vi "state name updater.vi"(1 "State Names":string[](array[string]), 2 "State Settings in":T1[][](array[typedef]) {"valve cycle time" min=0.2 step=0.1 format="%.2f"; "flow division"."5" min=0.0 max=1.0 step=0.01 format="%.3f"; "flow division"."4" min=0.0 max=1.0 step=0.01 format="%.3f"; "flow division"."3" min=0.0 max=1.0 step=0.01 format="%.3f"; "flow division"."2" min=0.0 max=1.0 step=0.01 format="%.3f"; "flow division"."1" min=0.0 max=1.0 step=0.01 format="%.3f"; "flow rate" format="%.3f"}) -> (0 "State Settings out":T1[][](array[typedef]) {"valve cycle time" min=0.2 step=0.1 format="%.2f"; "flow division"."5" min=0.0 max=1.0 step=0.01 format="%.3f"; "flow division"."4" min=0.0 max=1.0 step=0.01 format="%.3f"; "flow division"."3" min=0.0 max=1.0 step=0.01 format="%.3f"; "flow division"."2" min=0.0 max=1.0 step=0.01 format="%.3f"; "flow division"."1" min=0.0 max=1.0 step=0.01 format="%.3f"; "flow rate" format="%.3f"})   [LabVIEW 2012]
uses:
  State Setting.ctl
  Stamp/Switch settings vertical.ctl
  flow fraction.ctl
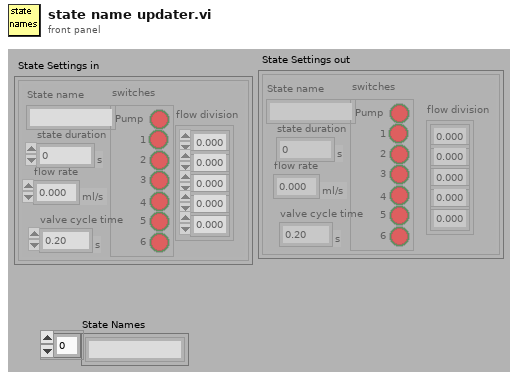
[diagram p1: front panel]
types:
  T1 = typedef "State Setting.ctl" = cluster{"switches":T2, "flow rate":dbl[unit], "flow division":cluster{"1":T3, "2":T3, "3":T3, "4":T3, "5":T3}, "State name":string, "state duration":dbl[unit], "valve cycle time":dbl[unit]}
  T2 = typedef "Switch settings vertical.ctl" = cluster{"Pump":bool, "1":bool, "2":bool, "3":bool, "4":bool, "5":bool, "6":bool}
  T3 = typedef "flow fraction.ctl" = dbl
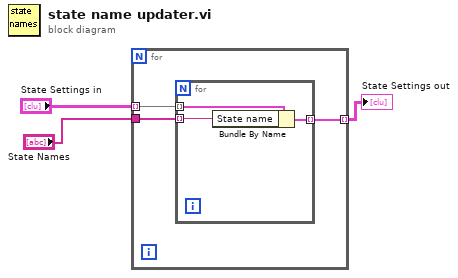
[diagram p0: block diagram]
diagram:
  n1 = for {
    tunnel: "State Settings in" -> [w6] mode=indexing
    tunnel: "State Names" -> [w5]
    tunnel: [w4] -> w1 mode=indexing
    n2 = for {
      tunnel: w6 -> [w9] mode=indexing
      tunnel: w5 -> [w8] mode=indexing
      tunnel: [w7] -> w4 mode=indexing
      n3 = Bundle By Name(cluster=w9, "State name"=w8) -> (w7:T1)
    }
  }
  "State Settings out" <- w1
